vi "Process.vi"(8 "error in":errorcluster, 11 "Instrument.Framework-Template in":refnum<class "Instrument.Framework-Template.lvclass">) -> (0 "error out":errorcluster, 3 "Instrument.Framework-Template out":refnum<class "Instrument.Framework-Template.lvclass">)   [LabVIEW 2019, in "Instrument.Framework-Template.lvclass"]
doc: "---------------------------------------------------------------\nJKI State Machine Objects™\nhttp://jki.net/state-machine-objects/\nCopyright (C) 2005-2015, JKI <info@jki.net>\nALL RIGHTS RESERVED"
uses:
  Instrument.Framework-Template.lvclass
  <userlib>/LevyLab/Instrument Framework/Instrument/Instrument.lvclass
  <userlib>/LevyLab/RemoteControl/RemoteControl/Typedefs/Message--Cluster.ctl
  <userlib>/LevyLab/RemoteControl/RemoteControl/RemoteControl.lvclass
  Typedefs/PrivateEvents--Framework-Template.MessageToProcess.ctl
  C:/Program Files (x86)/National Instruments/LabVIEW 2019/user.lib/LevyLab/Instrument Framework/Instrument Types/SCPI/Instrument.SCPI.lvclass
  C:/Program Files (x86)/National Instruments/LabVIEW 2019/user.lib/LevyLab/Instrument Framework/Instrument/Instrument.lvclass
  C:/Program Files (x86)/National Instruments/LabVIEW 2019/vi.lib/JKI/JKI SMO/SMO/SMO.lvclass
  <userlib>/LevyLab/Debug/Debug.lvlib
  <userlib>/LevyLab/Instrument Framework/Instrument/API/Instrument.sendMessageToProcess (variant).vi
  <vilib>/JKI/JKI SMO/SMO/SMO.lvclass
  <userlib>/LevyLab/Instrument Framework/Instrument Types/SCPI/Instrument.SCPI.lvclass
panel:
  out "Status":string
  out "State History":string
  # "Instrument.Framework-Template"
  # "Framework-Template"
  # "For instructions on how to use the JKI State Machine Objects, examples and video tutorials, visit:\nhttp://jki.net/state-machine-objects/\n\nJKI State Machine Objects™\nhttp://jki.net/state-machine-objects/\nCopyright (C) 2005-2015, JKI <info@jki.net>\nALL RIGHTS RESERVED"
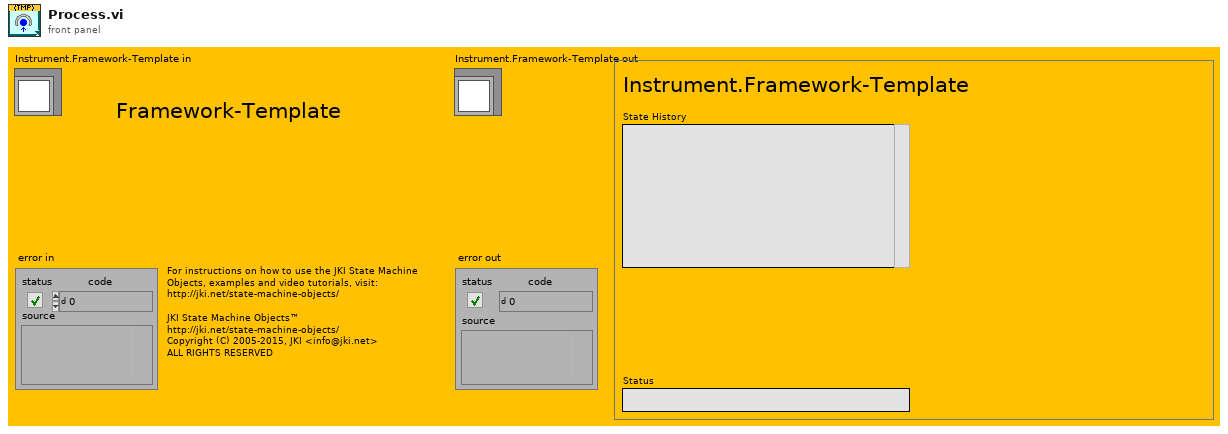
[diagram p1: front panel]
types:
  T1 = enum32{"invalid app kind", "Development System", "Run Time System", "Student Edition", "Embedded LabVIEW", "Evaluation", "Custom"}
  T2 = enum32{"Invalid", "Standard", "Closed", "Hidden", "Minimized", "Maximized"}
  T3 = typedef "RemoteControl.lvclass/Message--Cluster.ctl" = cluster{"Command":string, "Data":variant, "ID":string}
  T4 = typedef "Instrument.Framework-Template.lvclass/PrivateEvents--Framework-Template.MessageToProcess.ctl" = cluster{"Message":T5}
  T5 = typedef "RemoteControl.lvlib/RemoteControl.lvclass/Message--Cluster.ctl" = cluster{"Command":string, "Data":variant, "ID":string}
  T6 = cluster{"Core":cluster{"Current VI Reference":refnum<vi>, "Close Panel on Exit?":bool, "Last Error":cluster{"error":errorcluster, "previous state":string, "remaining states":string}, "Shutdown?":bool}, "SelfRef":refnum<class "Instrument.Framework-Template.lvclass">, "HAL":refnum<class "HAL.lvclass">, "Running Step":i32, "sequence":string[], "MessageToProcess":T4, "UI Behavior":string, "wait":u32}
  T7 = cluster{"Current VI Reference":refnum<vi>, "Close Panel on Exit?":bool, "Last Error":cluster{"error":errorcluster, "previous state":string, "remaining states":string}, "Shutdown?":bool}
  T8 = typedef "Debug.lvlib/Attribute.Debug.lvclass/DebugBehavior.ctl" = enum16{"Normal", "Debug"}
  T9 = typedef "SMO.lvclass/Protected Events.ctl" = cluster{"StopProcesses":refnum<user-event>, "AbortProcesses":refnum<user-event>, "Config Changed":refnum<user-event>, "Dependency":refnum<user-event>}
  T10 = typedef "Instrument.Framework-Template.lvclass/Instrument.Framework-Template.getAll--Cluster.ctl" = cluster{"Levy 1":dbl, "Logger SMO":dbl, "SMO Boolean":bool, "SMO String":string}
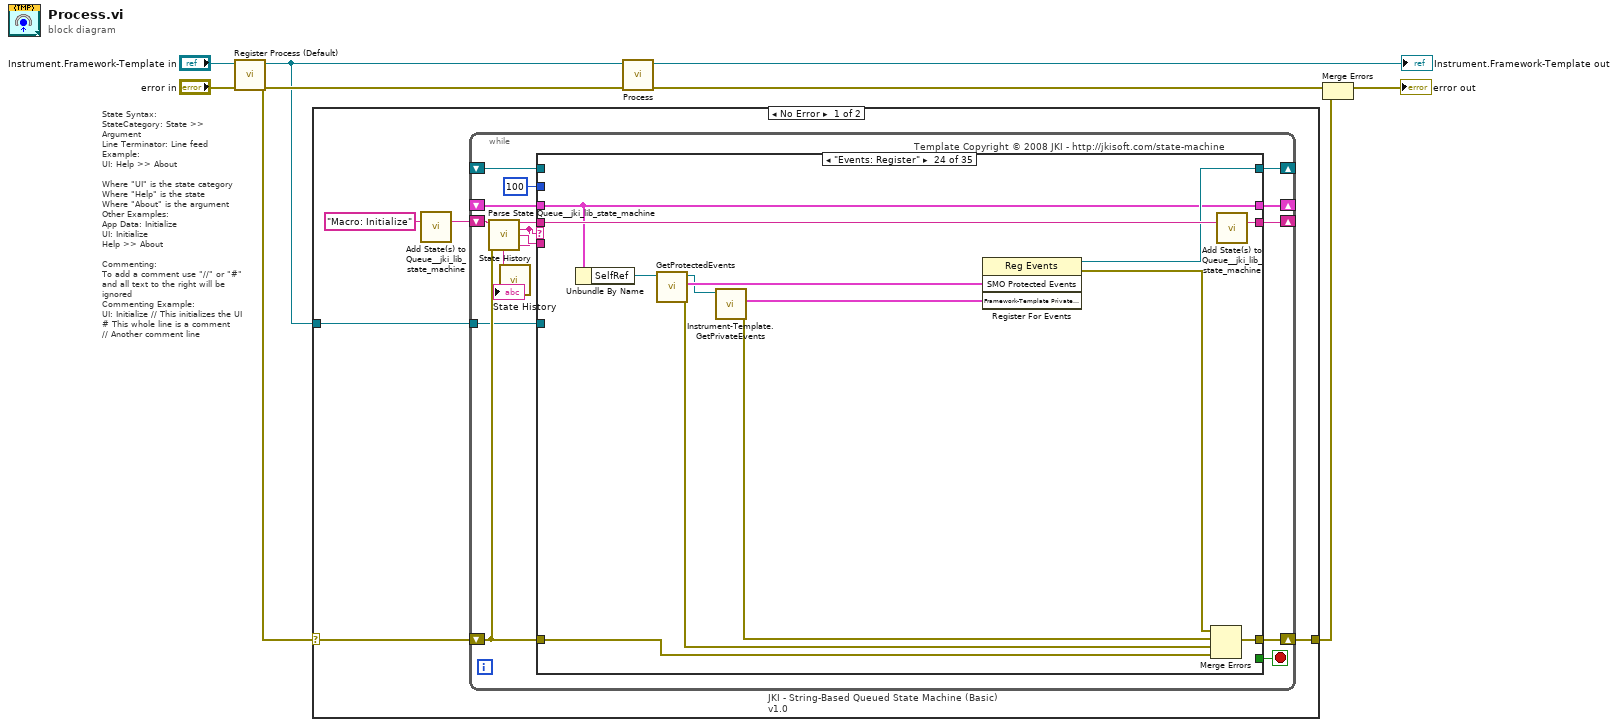
[diagram p0: block diagram]
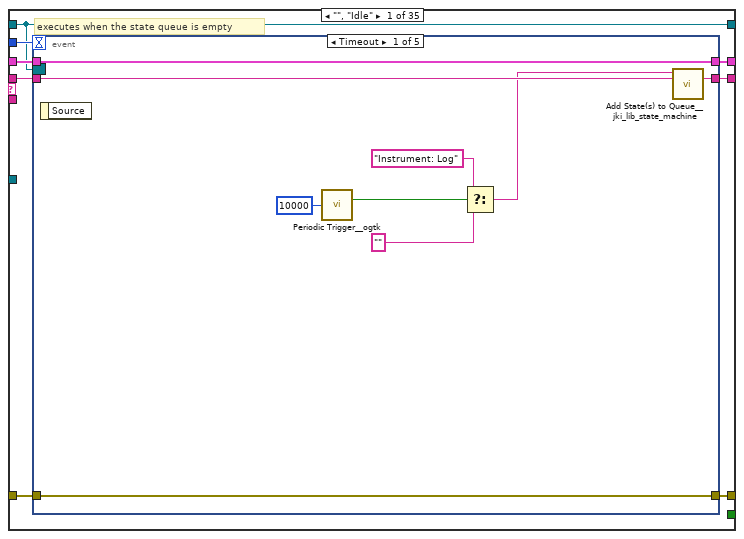
[diagram p2: hidden frame]
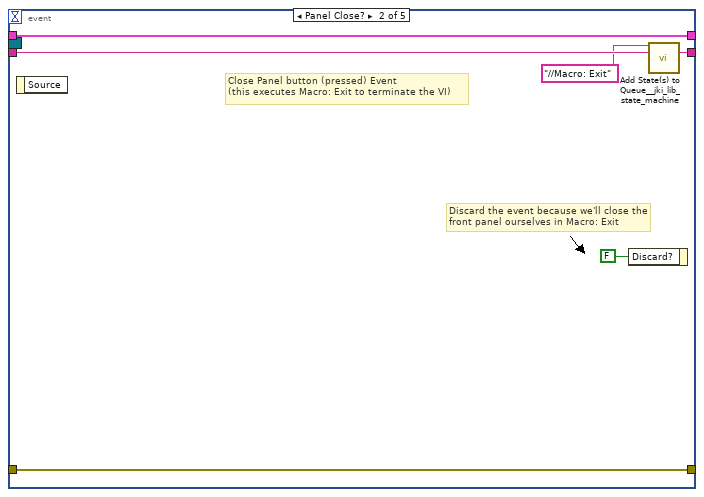
[diagram p3: hidden frame]
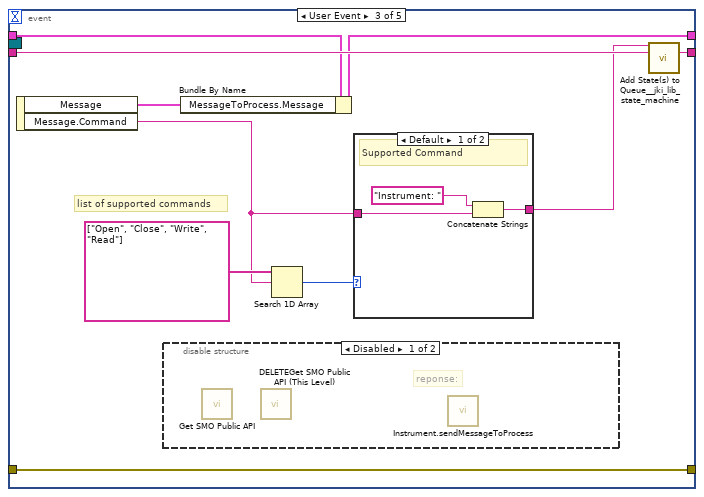
[diagram p4: hidden frame]
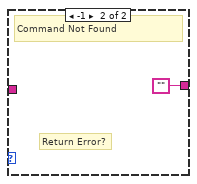
[diagram p6: hidden frame]
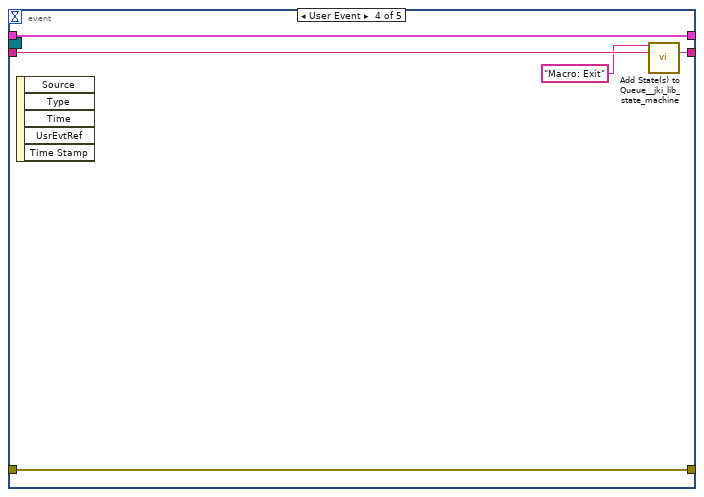
[diagram p7: hidden frame]
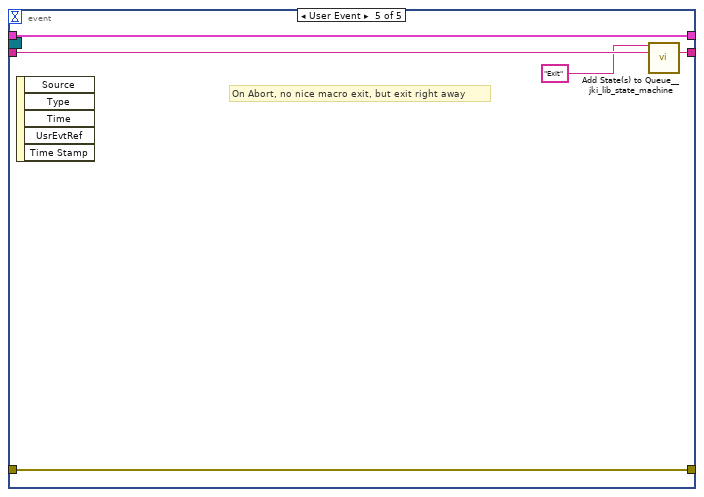
[diagram p8: hidden frame]
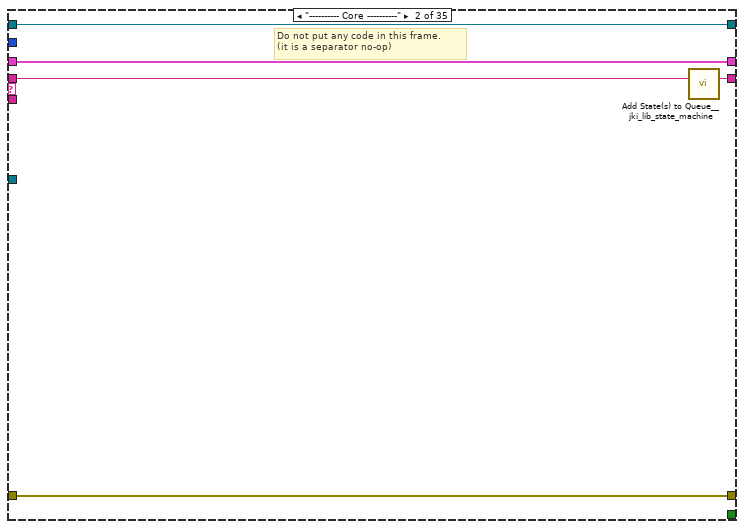
[diagram p9: hidden frame]
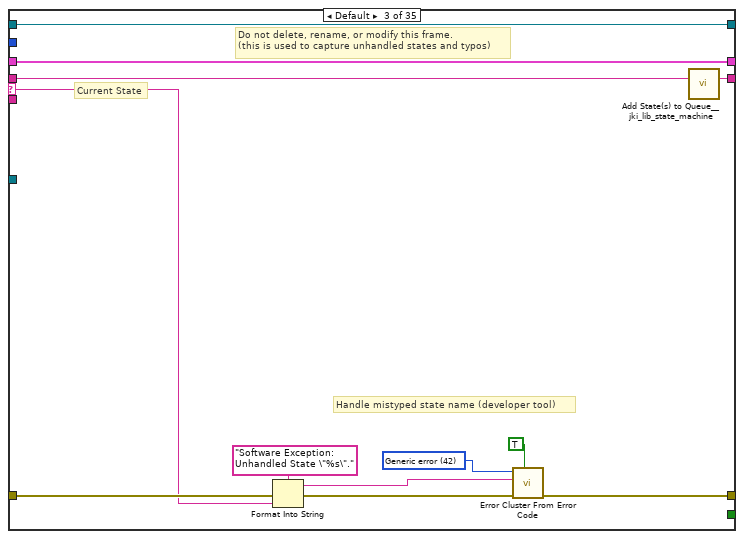
[diagram p10: hidden frame]
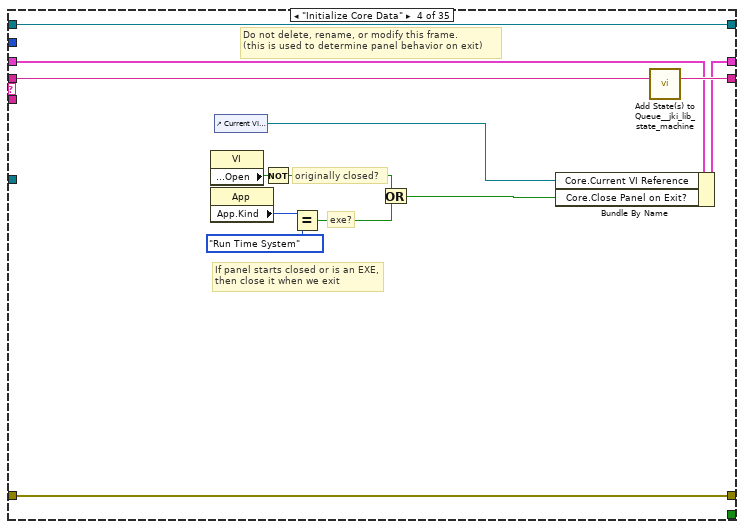
[diagram p11: hidden frame]
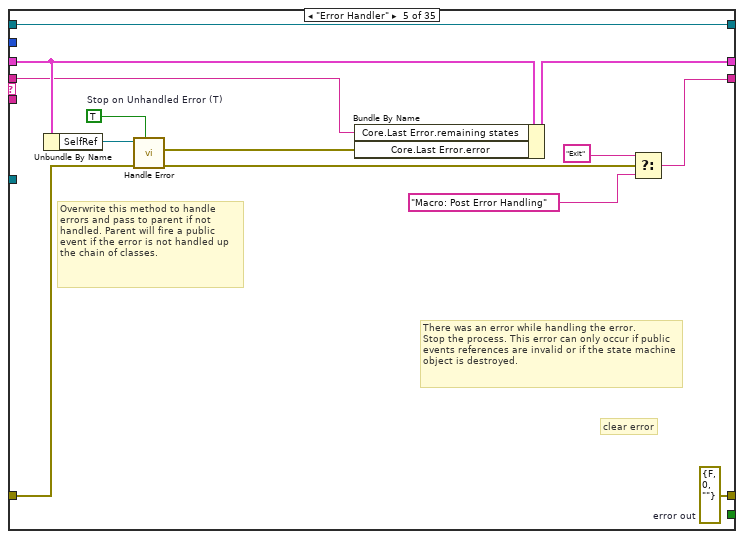
[diagram p12: hidden frame]
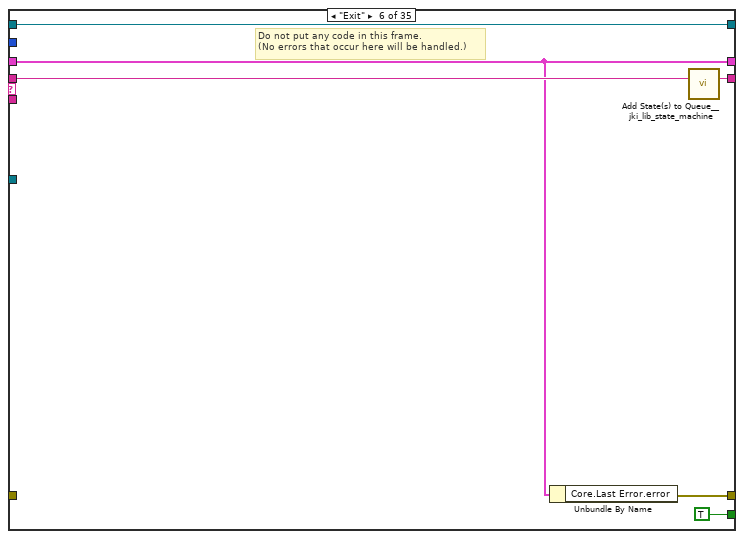
[diagram p13: hidden frame]
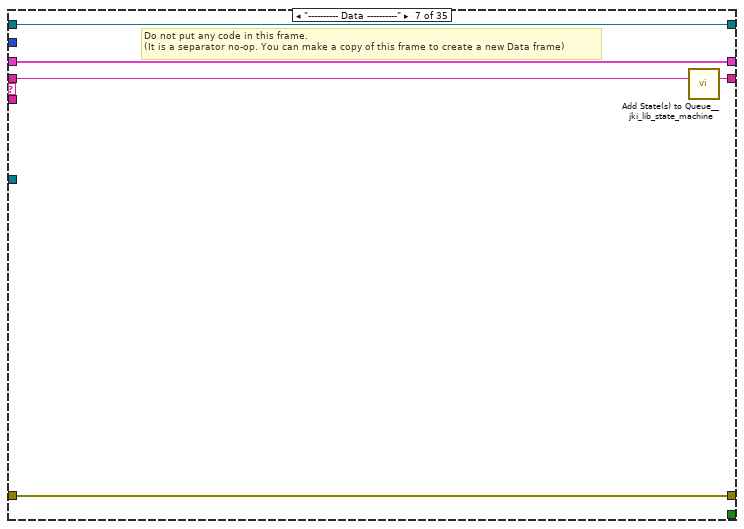
[diagram p14: hidden frame]
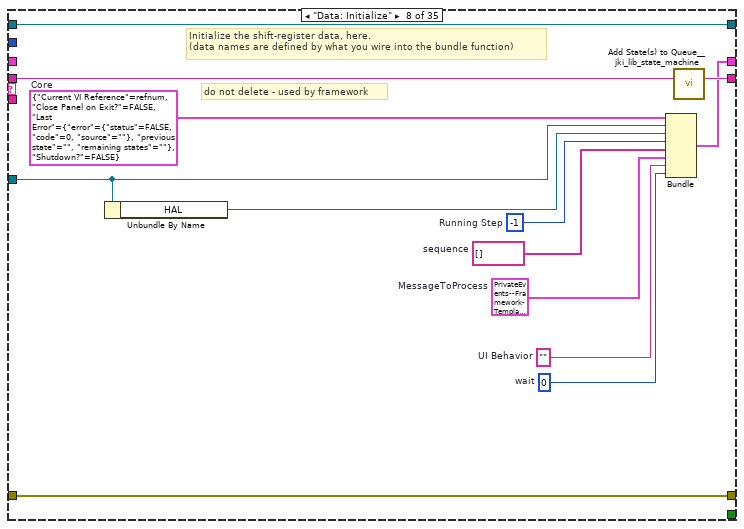
[diagram p15: hidden frame]
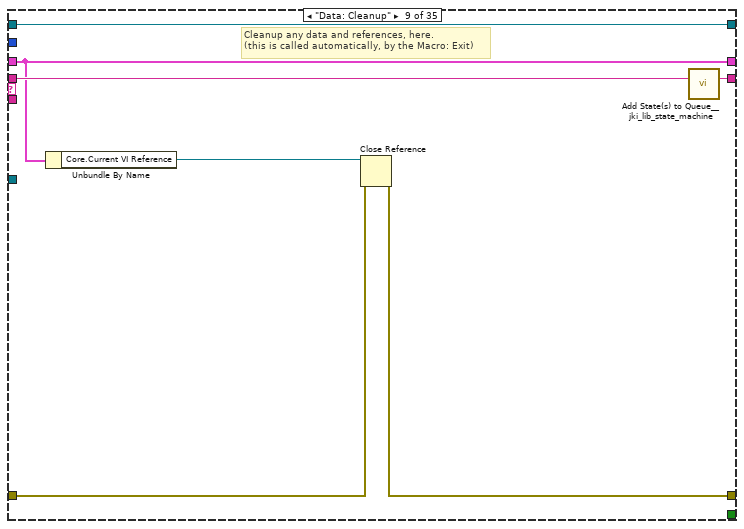
[diagram p16: hidden frame]
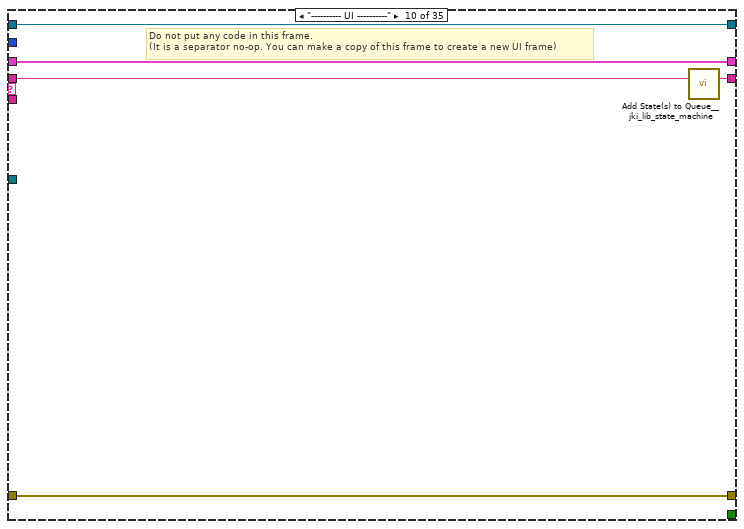
[diagram p17: hidden frame]
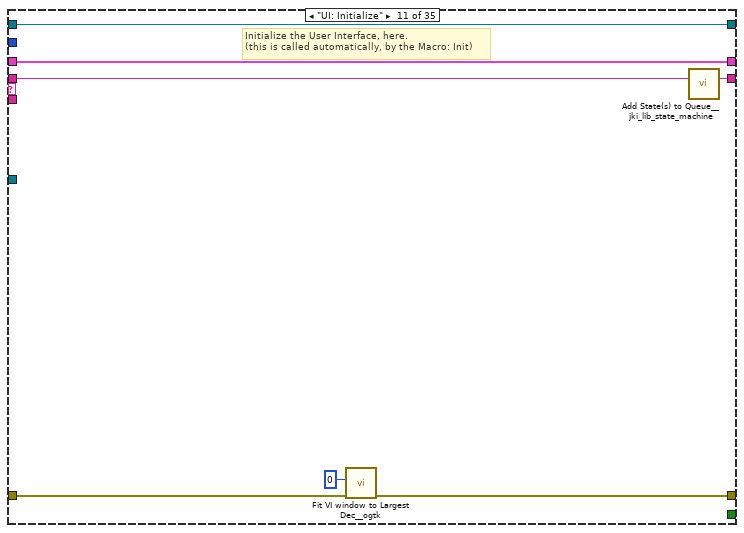
[diagram p18: hidden frame]
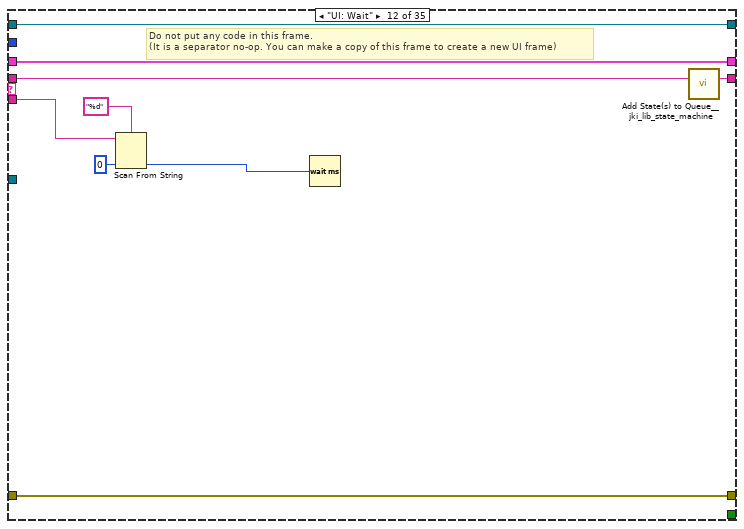
[diagram p19: hidden frame]
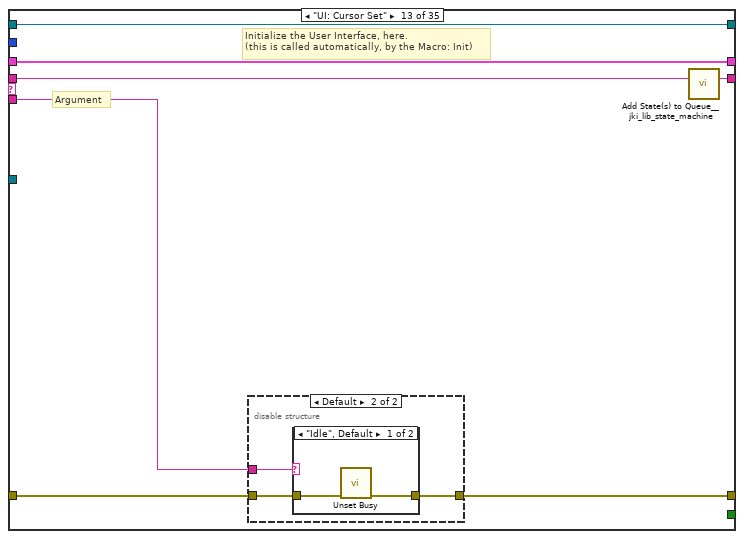
[diagram p20: hidden frame]
diagram:
  # "State Syntax:\nStateCategory: State >> Argument\nLine Terminator: Line feed\nExample:\nUI: Help >> About\n\nWhere \"UI\" is the state category\nWhere \"Help\" is the state\nWhere \"About\" is the argument\nOther Examples:\nApp Data: Initialize\nUI: Initialize\nHelp >> About\n\nCommenting:\nTo add a comment use \"//\" or \"#\" and all text to the right will be ignored\nCommenting Example:\nUI: Initialize // This initializes the UI\n# This whole line is a comment\n// Another comment line"
  n1 = call <vilib>:"Register Process (Default).vi"("error in (no error)"="error in", "SMO"="Instrument.Framework-Template in") -> ("error out"=w5:errorcluster, "SelfRef"=w4:refnum<class "Instrument.Framework-Template.lvclass">)  [unwired: 8 in]
  n2 = case shown="No Error" w5 {
    selector: w5 -> [w10 w455]
    tunnel: w4 -> [w11 _]
    tunnel: [w9 w455] -> w1
    frame No Error {
      n3 = call <vilib>:"Add State(s) to Queue__jki_lib_state_machine.vi"("State(s) in (\"\")"="Macro: Initialize") -> ("States Out"=w13:string)  [unwired: 14 in]
      n4 = while "JKI - String-Based Queued State Machine (Basic) v1.0" {
        shift-right: [w22] -> _
        shift-left: _ -> [w21]
        shift-right: [w25] -> w9
        shift-left: w10 -> [w19]
        shift-right: [w24] -> _
        shift-left: w13 -> [w26]
        tunnel: w11 -> [w18]
        shift-right: [w17] -> _
        shift-left: _ -> [w16]
        stop <- w23 stop-if-true
        # "Template Copyright © 2008 JKI - http://jkisoft.com/state-machine"
        n5 = call <vilib>:"Parse State Queue__jki_lib_state_machine.vi"("State Queue"=w26, "Error In (no error)"=w19) -> ("Remaining States"=w28:string, "Current State"=w15:string, "Arguments"=w27:string)  [unwired: 11 in]
        n6 = call <userlib>:"State History.vi"("Current State"=w15) -> ("History"=→"State History":string)  [unwired: 10 in]
        n7 = case shown="\"Events: Register\"" w15 {
          selector: w15 -> [_ _ w82 _ _ _ _ _ _ _ _ _ _ _ _ _ _ _ _ _ _ _ _ _ _ _ _ _ _ _ _ _ _ _ _]
          tunnel: w28 -> [w36 w80 w86 w105 w110 w124 w129 w142 w149 w154 w161 w170 w177 w193 w225 w234 w246 w267 w282 w304 w309 w320 w325 w338 w344 w352 w361 w370 w380 w389 w404 w424 w429 w435 w454]
          tunnel: w27 -> [_ _ _ _ _ _ _ _ _ _ _ w162 w171 w187 _ _ _ _ _ _ _ _ _ _ _ _ _ _ _ _ _ _ _ w430 w438]
          tunnel: w21 -> [w34 w77 w84 w96 w114 w120 w126 _ w144 w151 w159 w167 w175 w189 w222 w231 w236 w257 w271 w289 w306 w317 w322 w331 w342 w347 w357 w366 w376 w385 w400 w420 w425 w431 w444]
          tunnel: [w33 w78 w88 w102 w115 w119 w127 w132 w145 w152 w156 w168 w172 w190 w223 w226 w244 w265 w270 w292 w307 w311 w323 w334 w340 w349 w353 w365 w375 w384 w394 w418 w426 w432 w446] -> w25
          tunnel: w19 -> [w32 w78 w87 w102 w116 _ w127 w132 w146 w152 w155 w168 w173 w191 w223 w226 w244 w265 w269 w292 w307 w312 w323 w328 w340 w349 w356 w364 w374 w383 w398 w413 w426 w432 w440]
          tunnel: [w35 w79 w85 w104 w106 w123 w128 w141 w148 w153 w160 w169 w176 w192 w224 w233 w245 w266 w281 w303 w308 w319 w324 w337 w343 w351 w360 w369 w379 w388 w403 w423 w428 w434 w453] -> w24
          tunnel: [_ _ _ _ _ TRUE _ _ _ _ _ _ _ _ _ _ _ _ _ _ _ _ _ _ _ _ _ _ _ _ _ _ _ _ _] -> w23
          tunnel: [w31 w77 w84 w103 w113 w120 w126 w140 w144 w151 w159 w167 w175 w189 w222 w231 w237 w258 w272 w290 w306 w317 w322 w331 w342 w348 w358 w367 w377 w386 w401 w421 w425 w431 w443] -> w22
          tunnel: 100 ("Timeout") -> [w30 _ _ _ _ _ _ _ _ _ _ _ _ _ _ _ _ _ _ _ _ _ _ _ _ _ _ _ _ _ _ _ _ _ _]
          tunnel: w18 -> [_ _ _ _ _ _ _ w133 _ _ _ _ _ _ _ _ _ _ _ _ _ _ _ _ _ _ _ _ _ _ _ _ _ _ _]
          tunnel: [w29 w76 w81 w93 w118 w121 w125 w139 w143 w150 w158 w166 w174 w186 w221 w232 w243 w264 w280 w298 w305 w318 w321 w336 w341 w350 w359 w368 w378 w387 w402 w422 w427 w433 w452] -> w17
          tunnel: w16 -> [w29 w76 w81 w93 w118 w121 w125 w139 w143 w150 w158 w166 w174 w186 w221 w232 w243 w264 w280 w298 w305 w318 w321 _ w341 w350 w359 w368 w378 w387 w402 w422 w427 w433 w452]
          frame "", "Idle" {
            # "executes when the state queue is empty"
            n8 = event shown="[0] Timeout" {
              selector: w29 -> [_ _ _ _ _]
              dyn-events: _ -> [_ _ _ _ _]
              timeout: w30 -> [_ _ _ _ _]
              tunnel: w36 -> [w45 w51 w61 w70 w75]
              tunnel: [w44 w50 w60 w69 w74] -> w35
              tunnel: w34 -> [w42 w48 w53 w67 w72]
              tunnel: [w43 w49 w59 w68 w73] -> w33
              tunnel: w32 -> [w43 w49 w59 w68 w73]
              tunnel: [w42 w48 w54 w67 w72] -> w31
              event Timeout {
                n9 = event-data() -> ()  [unwired: 1 in, 1 out]
                n10 = call <userlib>:"Periodic Trigger__ogtk.vi"("time (ms)"=u32 10000) -> ("Triggered"=w39:bool)  [unwired: 12 in, 2 out]
                n11 = Select(t="Instrument: Log", s=w39, f="") -> (s? t:f=w40:string)
                n12 = call <vilib>:"Add State(s) to Queue__jki_lib_state_machine.vi"("State(s) in Front (\"\")"=w40, "State(s) in (\"\")"=w45) -> ("States Out"=w44:string)  [unwired: 13 in]
              }
              event Panel Close? {
                # "Discard the event because we'll close the front panel ourselves in Macro: Exit"
                # "Close Panel button (pressed) Event\n(this executes Macro: Exit to terminate the VI)"
                n13 = event-data() -> ()  [unwired: 1 in, 1 out]
                n14 = event-data("Discard?"=FALSE) -> ()  [unwired: 1 in, 1 out]
                n15 = call <vilib>:"Add State(s) to Queue__jki_lib_state_machine.vi"("State(s) in Front (\"\")"="//Macro: Exit", "State(s) in (\"\")"=w51) -> ("States Out"=w50:string)  [unwired: 13 in]
              }
              event User Event {
                # "list of supported commands"
                n16 = event-data() -> ("Message"=w52:T3, "Message.Command"=w55:string)  [unwired: 1 in]
                n17 = disable-structure shown="Disabled" {
                  frame Disabled {
                    # "reponse:"
                    n18 = call-dynamic "Get SMO Public API.vi"() -> ()  [unwired: 9 in, 3 out]
                    n19 = call-dynamic "DELETEGet SMO Public API (This Level).vi"() -> ()  [unwired: 9 in, 3 out]
                    n20 = call-poly <userlib>:"Instrument.sendMessageToProcess.vi"() -> ()  [unwired: 10 in, 2 out]
                  }
                  frame Enabled {
                  }
                }
                n21 = Bundle By Name(cluster=w53, "MessageToProcess.Message"=w52) -> (w54:T6)
                n22 = Search 1D Array(1D array=string[] ["Open", "Close", "Write", "Read"], element=w55) -> (index of element=w58:i32)  [unwired: 1 in]
                n23 = case shown="Default" w58 {
                  tunnel: [w64 ""] -> w56
                  tunnel: w55 -> [w63 _]
                  frame Default {
                    # "Supported Command"
                    n24 = Concatenate Strings("Instrument: ", w63) -> (w64:string)
                  }
                  frame -1 {
                    # "Return Error?"
                    # "Command Not Found"
                  }
                }
                n25 = call <vilib>:"Add State(s) to Queue__jki_lib_state_machine.vi"("State(s) in Front (\"\")"=w56, "State(s) in (\"\")"=w61) -> ("States Out"=w60:string)  [unwired: 13 in]
              }
              event User Event {
                n26 = event-data() -> ()  [unwired: 1 in, 5 out]
                n27 = call <vilib>:"Add State(s) to Queue__jki_lib_state_machine.vi"("State(s) in Front (\"\")"="Macro: Exit", "State(s) in (\"\")"=w70) -> ("States Out"=w69:string)  [unwired: 13 in]
              }
              event User Event {
                # "On Abort, no nice macro exit, but exit right away"
                n28 = event-data() -> ()  [unwired: 1 in, 5 out]
                n29 = call <vilib>:"Add State(s) to Queue__jki_lib_state_machine.vi"("State(s) in Front (\"\")"="Exit", "State(s) in (\"\")"=w75) -> ("States Out"=w74:string)  [unwired: 13 in]
              }
            }
          }
          frame "---------- Core ----------" {
            # "Do not put any code in this frame.\n(it is a separator no-op)"
            n30 = call <vilib>:"Add State(s) to Queue__jki_lib_state_machine.vi"("State(s) in (\"\")"=w80) -> ("States Out"=w79:string)  [unwired: 14 in]
          }
          frame Default {
            w91 = 42 items=["No error", "Argument error", "Memory is full", "Out of zone", "End of file", "File already open", "Generic file I/O error", "File not found", "File permission error", "Disk is full", "Duplicate path", "Too many files open", "System feature not enabled", "Resource file not found", "Cannot add resource", "Resource not found", "Image not found", "Image memory error", "Pen does not exist", "Config type invalid", "Config token not found", "Config parse error", "Config memory error", "Bad external code format", "Bad external code offset", "External code not present", "Null window", "Destroy window error", "Null menu", "Print aborted", "Bad print record", "Print driver error", "Windows error during printing", "Memory error during printing", "Print dialog error", "Generic print error", "Invalid device refnum", "Device not found", "Device parameter error", "Device unit error", "Cannot open device", "Device call aborted", "Generic error", "Cancelled by user", "Object ID too low", "Object ID too high", "Object not in heap", "Unknown heap", "Unknown object (invalid DefProc)", "Unknown object (DefProc not in table)", "Message out of range", "Invalid (null) method", "Unknown message", "Manager call not supported", "Bad address", "Network operation in progress", "Network operation timed out", "Connection is busy", "Network attribute not supported", "Network error", "Address in use", "System out of memory", "Connection aborted", "Connection refused", "Not connected", "Already connected", "Connection closed", "Initialization error (interapplication manager)", "Bad occurrence", "Wait on unbound occurrence handler", "Occurrence queue overflow", "Datalog type conflict", "Unused", "Unrecognized type (interapplication manager)", "Memory corrupt", "Failed to make temporary DLL", "Old CIN version", "Drag socket not found", "Failed to load drop-object", "Failed to register OLE object", "Failed to release OLE object", "Format specifier type mismatch", "Unknown format specifier", "Too few format specifiers", "Too many format specifiers", "Scan failed", "Newer CIN version", "Error converting to variant", "Runtime menu error", "Password tampered", "Variant attribute not found", "Incompatible variant data type", "Event data is not available", "Event Store is not present", "Occurrence is not found", "Event Queue is not created", "Event info is not available", "Refnum passed is NULL", "Error retrieving Class GUID", "Error retrieving CoClass GUID", "Error retrieving TypeLib GUID.", "Bad built application magic bytes.", "Specific driver is different from the specific driver associated with the Logical Name.", "There is no session opened to the class driver.", "Max Error", "MAX - Error with config objects", "MAX - Error loading configuration", "MAX - Group not supported"]
            # "Current State"
            # "Do not delete, rename, or modify this frame.\n(this is used to capture unhandled states and typos)"
            # "Handle mistyped state name (developer tool)"
            n31 = Format Into String(format string="Software Exception: Unhandled State \"%s\"." ("message"), error in=w87, w82) -> (resulting string=w90:string, error out=w89:errorcluster)  [unwired: 1 in]
            n32 = call <vilib>:"Error Cluster From Error Code.vi"("show call chain? (False)"=TRUE, "error in (no error)"=w89, "error message (\"\")"=w90, "error code (0)"=w91) -> ("error out"=w88:errorcluster)  [unwired: 5 in]
            n33 = call <vilib>:"Add State(s) to Queue__jki_lib_state_machine.vi"("State(s) in (\"\")"=w86) -> ("States Out"=w85:string)  [unwired: 14 in]
          }
          frame "Initialize Core Data" {
            # "Do not delete, rename, or modify this frame.\n(this is used to determine panel behavior on exit)"
            # "originally closed?"
            # "exe?"
            # "If panel starts closed or is an EXE, then close it when we exit"
            n34 = property class="VI"() -> ("Front Panel.Open"=w101:bool)  [unwired: 2 in, 2 out]
            n35 = property class="App"() -> ("App.Kind"=w100:T1)  [unwired: 2 in, 2 out]
            n36 = control-ref of="Current VI Reference"() -> (w94:refnum<vi>)
            n37 = Not(x=w101) -> (.not. x?=w98:bool)
            n38 = Equal?(x=w100, y=T1."Run Time System" ("Application:Kind")) -> (x = y?=w97:bool)
            n39 = Or(x=w98, y=w97) -> (x .or. y?=w95:bool)
            n40 = Bundle By Name(cluster=w96, "Core.Current VI Reference"=w94, "Core.Close Panel on Exit?"=w95) -> (w103:T6)
            n41 = call <vilib>:"Add State(s) to Queue__jki_lib_state_machine.vi"("State(s) in (\"\")"=w105) -> ("States Out"=w104:string)  [unwired: 14 in]
          }
          frame "Error Handler" {
            w111 = TRUE  # Stop on Unhandled Error (T)
            w115 = errorcluster {"status"=FALSE, "code"=0, "source"=""}  # error out
            # "clear error"
            # "There was an error while handling the error.\nStop the process. This error can only occur if public events references are invalid or if the state machine object is destroyed."
            # "Overwrite this method to handle errors and pass to parent if not handled. Parent will fire a public event if the error is not handled up the chain of classes."
            n42 = Unbundle By Name(w114) -> ("SelfRef"=w117:refnum<class "Instrument.Framework-Template.lvclass">)
            n43 = call-dynamic "Handle Error.vi"("Stop on Unhandled Error (T)"=w111, "error in"=w116, "SMO"=w117) -> ("handling error"=w107:errorcluster, "Unhandled error"=w112:errorcluster)  [unwired: 6 in, 1 out]
            n44 = Bundle By Name(cluster=w114, "Core.Last Error.remaining states"=w110, "Core.Last Error.error"=w112) -> (w113:T6)
            n45 = Select(t="Exit", s=w107, f="Macro: Post Error Handling") -> (s? t:f=w106:string)
          }
          frame "Exit" {
            # "Do not put any code in this frame.\n(No errors that occur here will be handled.)"
            n46 = Unbundle By Name(w120) -> ("Core.Last Error.error"=w119:errorcluster)
            n47 = call <vilib>:"Add State(s) to Queue__jki_lib_state_machine.vi"("State(s) in (\"\")"=w124) -> ("States Out"=w123:string)  [unwired: 14 in]
          }
          frame "---------- Data ----------" {
            # "Do not put any code in this frame.\n(It is a separator no-op. You can make a copy of this frame to create a new Data frame)"
            n48 = call <vilib>:"Add State(s) to Queue__jki_lib_state_machine.vi"("State(s) in (\"\")"=w129) -> ("States Out"=w128:string)  [unwired: 14 in]
          }
          frame "Data: Initialize" {
            w130 = u32 0  # wait
            w131 = ""  # UI Behavior
            w135 = T4 {"Message"={"Command"="", "Data"=variant(string ""), "ID"=""}}  # MessageToProcess
            w136 = string[] []  # sequence
            w137 = -1  # Running Step
            w138 = T7 {"Current VI Reference"=refnum, "Close Panel on Exit?"=FALSE, "Last Error"={"error"={"status"=FALSE, "code"=0, "source"=""}, "previous state"="", "remaining states"=""}, "Shutdown?"=FALSE}  # Core
            # "do not delete - used by framework"
            # "Initialize the shift-register data, here.\n(data names are defined by what you wire into the bundle function)"
            n49 = Unbundle By Name(w133) -> ("HAL"=w134:refnum<class "HAL.lvclass">)
            n50 = Bundle("Core"=w138, "SelfRef"=w133, "HAL"=w134, "Running Step"=w137, "sequence"=w136, "MessageToProcess"=w135, "UI Behavior"=w131, "wait"=w130) -> (w140:T6)  [unwired: 1 in]
            n51 = call <vilib>:"Add State(s) to Queue__jki_lib_state_machine.vi"("State(s) in (\"\")"=w142) -> ("States Out"=w141:string)  [unwired: 14 in]
          }
          frame "Data: Cleanup" {
            # "Cleanup any data and references, here.\n(this is called automatically, by the Macro: Exit)"
            n52 = Unbundle By Name(w144) -> ("Core.Current VI Reference"=w147:refnum<vi>)
            n53 = Close Reference(reference=w147, error in (no error)=w146) -> (error out=w145:errorcluster)
            n54 = call <vilib>:"Add State(s) to Queue__jki_lib_state_machine.vi"("State(s) in (\"\")"=w149) -> ("States Out"=w148:string)  [unwired: 14 in]
          }
          frame "---------- UI ----------" {
            # "Do not put any code in this frame.\n(It is a separator no-op. You can make a copy of this frame to create a new UI frame)"
            n55 = call <vilib>:"Add State(s) to Queue__jki_lib_state_machine.vi"("State(s) in (\"\")"=w154) -> ("States Out"=w153:string)  [unwired: 14 in]
          }
          frame "UI: Initialize" {
            # "Initialize the User Interface, here.\n(this is called automatically, by the Macro: Init)"
            n56 = call <userlib>:"Fit VI window to Largest Dec__ogtk.vi"("error in (no error)"=w155, "border spacing (2 px)"=0) -> ("error out"=w156:errorcluster)  [unwired: 4 in, 1 out]
            n57 = call <vilib>:"Add State(s) to Queue__jki_lib_state_machine.vi"("State(s) in (\"\")"=w161) -> ("States Out"=w160:string)  [unwired: 14 in]
          }
          frame "UI: Wait" {
            # "Do not put any code in this frame.\n(It is a separator no-op. You can make a copy of this frame to create a new UI frame)"
            n58 = Scan From String(format string="%d", input string=w162, default 1=u32 0 ("default value 1")) -> (output 1=w163:u32)  [unwired: 2 in, 3 out]
            n59 = Wait (ms)(milliseconds to wait=w163) -> ()  [unwired: 1 out]
            n60 = call <vilib>:"Add State(s) to Queue__jki_lib_state_machine.vi"("State(s) in (\"\")"=w170) -> ("States Out"=w169:string)  [unwired: 14 in]
          }
          frame "UI: Cursor Set" {
            # "Argument"
            # "Initialize the User Interface, here.\n(this is called automatically, by the Macro: Init)"
            n61 = disable-structure shown="Default" {
              disable-tunnel: w173 -> [w178 w181]
              disable-tunnel: [w178 w180] -> w172
              disable-tunnel: w171 -> [_ w179]
              frame condition #0 {
              }
              frame condition #1 (active) {
                n62 = case shown="\"Idle\", Default" w179 {
                  tunnel: w181 -> [w183 w185]
                  tunnel: [w182 w184] -> w180
                  frame "Idle", Default {
                    n63 = call <vilib>:"Unset Busy.vi"("error in (no error)"=w183) -> ("error out"=w182:errorcluster)  [unwired: 10 in]
                  }
                  frame "Busy" {
                    n64 = call <vilib>:"Set Busy.vi"("error in (no error)"=w185) -> ("error out"=w184:errorcluster)  [unwired: 9 in, 1 out]
                  }
                }
              }
            }
            n65 = call <vilib>:"Add State(s) to Queue__jki_lib_state_machine.vi"("State(s) in (\"\")"=w177) -> ("States Out"=w176:string)  [unwired: 14 in]
          }
          frame "UI: Front Panel State" {
            # "Argument"
            # "Set Front Panel Open or Closed\n(Usage: \"UI: Front Panel State >> Open|Close\")"
            n66 = Unbundle By Name(w189) -> ("Core.Current VI Reference"=w188:refnum<vi>)
            n67 = disable-structure shown="TARGET_TYPE==RT" {
              disable-tunnel: w191 -> [w197 w220]
              disable-tunnel: [w196 w220] -> w190
              disable-tunnel: w188 -> [w195 _]
              disable-tunnel: w187 -> [w194 _]
              frame condition #0 (active) {
                n68 = case shown="\"Close\"" w194 {
                  tunnel: w197 -> [w201 w214]
                  tunnel: [w203 w215] -> w196
                  tunnel: w195 -> [w202 w212]
                  frame "Open", Default {
                    n69 = property class="VI"(reference=w202, error in=w201) -> (reference out=w199:refnum<vi>, error out=w200:errorcluster, "FP.State"=w198:T2)
                    n70 = case shown="\"Closed\"" w198 {
                      tunnel: [w206 w209] -> w203
                      tunnel: w200 -> [w205 w209]
                      tunnel: w199 -> [w204 _]
                      frame "Closed" {
                        n71 = invoke class="VI" method="FP.Open"(reference=w204, error in=w205, "Activate"=TRUE, "State"=T2."Standard") -> (error out=w206:errorcluster)  [unwired: 1 in, 4 out]
                      }
                      frame Default {
                      }
                    }
                  }
                  frame "Close" {
                    n72 = property class="VI"(reference=w212, error in=w214) -> (reference out=w211:refnum<vi>, error out=w213:errorcluster, "FP.State"=w210:T2)
                    n73 = case shown="Default" w210 {
                      tunnel: [w216 w219] -> w215
                      tunnel: w213 -> [w216 w218]
                      tunnel: w211 -> [_ w217]
                      frame "Invalid", "Closed" {
                      }
                      frame Default {
                        n74 = invoke class="VI" method="FP.Close"(reference=w217, error in=w218) -> (error out=w219:errorcluster)  [unwired: 1 in, 2 out]
                      }
                    }
                  }
                }
              }
              frame condition #1 {
              }
            }
            n75 = call <vilib>:"Add State(s) to Queue__jki_lib_state_machine.vi"("State(s) in (\"\")"=w193) -> ("States Out"=w192:string)  [unwired: 14 in]
          }
          frame "---------- Macro ----------" {
            # "Do not put any code in this frame.\n(It is a separator no-op. You can make a copy of this frame to create a new Macro frame)"
            n76 = call <vilib>:"Add State(s) to Queue__jki_lib_state_machine.vi"("State(s) in (\"\")"=w225) -> ("States Out"=w224:string)  [unwired: 14 in]
          }
          frame "Macro: Initialize" {
            # "Initialization Macro\n(This is called once, when the VI starts)"
            n77 = call <vilib>:"Add State(s) to Queue__jki_lib_state_machine.vi"("State(s) in Front (\"\")"="Data: Initialize\nInitialize Core Data\nEvents: Register", "State(s) in (\"\")"="Process: Sync", "State(s) at Back (\"\")"="UI: Initialize\nUI: Front Panel State >> Close\nInstrument: Open\nMacro: Debug") -> ("States Out"=w229:string)  [unwired: 12 in]
            n78 = call <vilib>:"Add State(s) to Queue__jki_lib_state_machine.vi"("State(s) in Front (\"\")"=w229, "State(s) in (\"\")"=w234) -> ("States Out"=w233:string)  [unwired: 13 in]
          }
          frame "Macro: Post Error Handling" {
            # "Clear Last Error?"
            n79 = Unbundle By Name(w236) -> ("Core.Last Error.remaining states"=w238:string, "Core.Shutdown?"=w239:bool)
            n80 = Unbundle By Name(w236) -> ("Core.Last Error.error"=w242:errorcluster)
            n81 = case shown="False" FALSE {
              tunnel: w242 -> [w250 _]
              tunnel: [w250 _] -> w241
              frame False {
              }
              frame True {
              }
            }
            n82 = case shown="False" w239 {
              tunnel: w238 -> [w247 w249]
              tunnel: [w247 w248] -> w235
              frame False {
                # "These are the remaining states (at the moment the error occured). States can be altered according to business logic."
                # "NOT SHUTTING DOWN"
              }
              frame True {
                # "Developer can decide to alter the states but should be aware that during the shutdown process, there are certain states that must be run for the SMO to properly shut itself (and this process) down. As such, one can add states to perform additional clean-ups, but should append the remaining state to be executed."
                # "SHUTTING DOWN"
                n83 = call <vilib>:"Add State(s) to Queue__jki_lib_state_machine.vi"("State(s) in (\"\")"=w249) -> ("States Out"=w248:string)  [unwired: 14 in]
              }
            }
            n84 = Bundle By Name(cluster=w236, "Core.Last Error.error"=w241) -> (w237:T6)
            n85 = call <vilib>:"Add State(s) to Queue__jki_lib_state_machine.vi"("State(s) in Front (\"\")"=w235, "State(s) in (\"\")"=w246) -> ("States Out"=w245:string)  [unwired: 13 in]
          }
          frame "Macro: Run Sequence" {
            # "0,1,2,3,4,"
            # "5"
            # "Do not put any code in this frame.\n(It is a separator no-op. You can make a copy of this frame to create a new Macro frame)"
            n86 = Unbundle By Name(w257) -> ("sequence"=w253:string[], "Running Step"=w251:i32)
            n87 = Array Size(array=w253) -> (size(s)=w263:i32)
            n88 = Index Array(array=w253, index=w251) -> (element=w252:string)
            n89 = Greater Or Equal?(x=w263, y=w251) -> (x >= y?=w255:bool)
            n90 = Select(t=-1 ("Running Step"), s=w255, f=w251) -> (s? t:f=w262:i32)
            n91 = Bundle By Name(cluster=w257, "Running Step"=w262) -> (w258:T6)
            n92 = Select(t="Sequence: Status >> ...", s=w255, f="Idle //Check Event Structure\nMacro: Run Sequence" ("State(s) at Back (\"\")")) -> (s? t:f=w254:string)
            n93 = call <vilib>:"Add State(s) to Queue__jki_lib_state_machine.vi"("State(s) in Front (\"\")"=w252, "State(s) at Back (\"\")"=w254) -> ("States Out"=w256:string)  [unwired: 13 in]
            n94 = call <vilib>:"Add State(s) to Queue__jki_lib_state_machine.vi"("State(s) in Front (\"\")"=w256, "State(s) in (\"\")"=w267) -> ("States Out"=w266:string)  [unwired: 13 in]
          }
          frame "Macro: Debug" {
            # "exe?"
            # "If pane is an EXE, then close it when we exit"
            # "Macro: Debug\n(get debug behavior, determine UI and determine shutdown behavior)"
            n95 = Unbundle By Name(w271) -> ("Core.Close Panel on Exit?"=w274:bool, "SelfRef"=w279:refnum<class "Instrument.Framework-Template.lvclass">)
            n96 = property class="App"() -> ("App.Kind"=w277:T1)  [unwired: 2 in, 2 out]
            n97 = Equal?(x=w277, y=T1."Run Time System" ("Application:Kind")) -> (x = y?=w273:bool)
            n98 = call <userlib>:"Get Debug Mode.vi"("error in (no error)"=w269, "SMO"=w279) -> ("error out"=w270:errorcluster, "Behavior"=w278:T8)  [unwired: 7 in, 1 out]
            n99 = case shown="\"Normal\", Default" w278 {
              tunnel: [w283 w285] -> w275
              tunnel: w274 -> [w283 _]
              tunnel: w273 -> [_ w287]
              tunnel: [_ "UI: Front Panel State >> Open\nUI: Wait >> 1000"] -> w268
              frame "Normal", Default {
                # "respect core.close"
              }
              frame "Debug" {
                # "keep panel open\nunless exe"
                n100 = Or(x=w287, y=FALSE) -> (x .or. y?=w285:bool)
              }
            }
            n101 = Bundle By Name(cluster=w271, "Core.Close Panel on Exit?"=w275) -> (w272:T6)
            n102 = call <vilib>:"Add State(s) to Queue__jki_lib_state_machine.vi"("State(s) in Front (\"\")"=w268, "State(s) in (\"\")"=w282) -> ("States Out"=w281:string)  [unwired: 13 in]
          }
          frame "Macro: Exit" {
            # "Exit Macro\n(This is called once, when the VI exits)"
            n103 = Unbundle By Name(w289) -> ("Core.Close Panel on Exit?"=w302:bool)
            n104 = Select(t="UI: Front Panel State >> Close", s=w302, f="") -> (s? t:f=w300:string)
            n105 = Bundle By Name(cluster=w289, "Core.Shutdown?"=TRUE) -> (w290:T6)
            n106 = call <vilib>:"Add State(s) to Queue__jki_lib_state_machine.vi"("State(s) in Front (\"\")"="Data: Cleanup\nEvents: Unregister", "State(s) in (\"\")"="Process: Sync", "State(s) at Back (\"\")"="Exit") -> ("States Out"=w295:string)  [unwired: 12 in]
            n107 = call <vilib>:"Add State(s) to Queue__jki_lib_state_machine.vi"("State(s) in Front (\"\")"="Instrument: Close", "State(s) in (\"\")"=w300, "State(s) at Back (\"\")"=w295) -> ("States Out"=w299:string)  [unwired: 12 in]
            n108 = call <vilib>:"Add State(s) to Queue__jki_lib_state_machine.vi"("State(s) in Front (\"\")"=w299, "State(s) in (\"\")"=w304) -> ("States Out"=w303:string)  [unwired: 13 in]
          }
          frame "---------- Process ----------" {
            # "Template Separator\n(You can make a copy of, or modify, this frame)"
            n109 = call <vilib>:"Add State(s) to Queue__jki_lib_state_machine.vi"("State(s) in (\"\")"=w309) -> ("States Out"=w308:string)  [unwired: 14 in]
          }
          frame "Process: Sync" {
            n110 = Unbundle By Name(w317) -> ("SelfRef"=w313:refnum<class "Instrument.Framework-Template.lvclass">)
            n111 = call <vilib>:"WaitOnProcessSync.vi"("error in (no error)"=w312, "SMO"=w313) -> ("error out"=w311:errorcluster, "Don't run?"=w316:bool)  [unwired: 7 in, 1 out]
            n112 = Select(t="Data: Cleanup\nEvents: Unregister\nExit", s=w316, f="") -> (s? t:f=w310:string)
            n113 = call <vilib>:"Add State(s) to Queue__jki_lib_state_machine.vi"("State(s) in Front (\"\")"=w310, "State(s) in (\"\")"=w320) -> ("States Out"=w319:string)  [unwired: 13 in]
          }
          frame "---------- Events ----------" {
            # "Template Separator\n(You can make a copy of, or modify, this frame)"
            n114 = call <vilib>:"Add State(s) to Queue__jki_lib_state_machine.vi"("State(s) in (\"\")"=w325) -> ("States Out"=w324:string)  [unwired: 14 in]
          }
          frame "Events: Register" {
            n115 = Unbundle By Name(w331) -> ("SelfRef"=w332:refnum<class "Instrument.Framework-Template.lvclass">)
            n116 = call <vilib>:"GetProtectedEvents.vi"("SMO"=w332) -> ("error out"=w330:errorcluster, "SMO Protected Events"=w335:T9, "SMO out"=w329:refnum<class "Instrument.Framework-Template.lvclass">)  [unwired: 8 in]
            n117 = call "Instrument-Template.GetPrivateEvents.vi"("Instrument.Framework-Template in"=w329) -> ("error out"=w326:errorcluster, "Framework-Template Private Events"=w327:cluster{"MessageToProcess":refnum<user-event>})  [unwired: 8 in, 1 out]
            n118 = register-events(w335, w327) -> (reference out=w336:refnum<event-registration>, error out=w333:errorcluster)  [unwired: 2 in]
            n119 = Merge Errors(w333, w326, w330, w328) -> (w334:errorcluster)
            n120 = call <vilib>:"Add State(s) to Queue__jki_lib_state_machine.vi"("State(s) in (\"\")"=w338) -> ("States Out"=w337:string)  [unwired: 14 in]
          }
          frame "Events: Unregister" {
            n121 = Unregister For Events(event registration refnum=w341, error in=w340) -> (error out=w339:errorcluster)
            n122 = call <vilib>:"Clear Errors.vi"("error in (no error)"=w339) -> ()  [unwired: 5 in, 2 out]
            n123 = call <vilib>:"Add State(s) to Queue__jki_lib_state_machine.vi"("State(s) in (\"\")"=w344) -> ("States Out"=w343:string)  [unwired: 14 in]
          }
          frame "---------- Instrument ----------" {
            n124 = Unbundle By Name(w347) -> ("SelfRef"=w345:refnum<class "Instrument.Framework-Template.lvclass">, "HAL"=w346:refnum<class "HAL.lvclass">)
            n125 = Bundle By Name(cluster=w347, "SelfRef"=w345, "HAL"=w346) -> (w348:T6)
            n126 = call <vilib>:"Add State(s) to Queue__jki_lib_state_machine.vi"("State(s) in (\"\")"=w352) -> ("States Out"=w351:string)  [unwired: 14 in]
          }
          frame "Instrument: Open" {
            n127 = Unbundle By Name(w357) -> ("SelfRef"=w355:refnum<class "Instrument.Framework-Template.lvclass">)
            n128 = call-dynamic "Open Hardware.vi"("error in (no error)"=w356, "Instrument in"=w355) -> ("error out"=w353:errorcluster, "Instrument out"=w354:refnum<class "Instrument.Framework-Template.lvclass">)  [unwired: 8 in]
            n129 = Bundle By Name(cluster=w357, "SelfRef"=w354) -> (w358:T6)
            n130 = call <vilib>:"Add State(s) to Queue__jki_lib_state_machine.vi"("State(s) in (\"\")"=w361) -> ("States Out"=w360:string)  [unwired: 14 in]
          }
          frame "Instrument: Write" {
            n131 = Unbundle By Name(w366) -> ("SelfRef"=w363:refnum<class "Instrument.Framework-Template.lvclass">)
            n132 = call-dynamic "Write Hardware.vi"("error in (no error)"=w364, "Instrument in"=w363) -> ("error out"=w365:errorcluster, "Instrument out"=w362:refnum<class "Instrument.Framework-Template.lvclass">)  [unwired: 8 in]
            n133 = Bundle By Name(cluster=w366, "SelfRef"=w362) -> (w367:T6)
            n134 = call <vilib>:"Add State(s) to Queue__jki_lib_state_machine.vi"("State(s) in (\"\")"=w370) -> ("States Out"=w369:string)  [unwired: 14 in]
          }
          frame "Instrument: Read" {
            n135 = Unbundle By Name(w376) -> ("SelfRef"=w372:refnum<class "Instrument.Framework-Template.lvclass">)
            n136 = call-dynamic "Read Hardware.vi"("error in (no error)"=w374, "Instrument in"=w372) -> ("error out"=w375:errorcluster, "response"=w373:string, "Instrument out"=w371:refnum<class "Instrument.Framework-Template.lvclass">)  [unwired: 7 in]
            n137 = Bundle By Name(cluster=w376, "SelfRef"=w371, "MessageToProcess.Message.Data"=w373) -> (w377:T6)
            n138 = call <vilib>:"Add State(s) to Queue__jki_lib_state_machine.vi"("State(s) in (\"\")"=w380) -> ("States Out"=w379:string)  [unwired: 14 in]
          }
          frame "Instrument: Close" {
            n139 = Unbundle By Name(w385) -> ("SelfRef"=w382:refnum<class "Instrument.Framework-Template.lvclass">)
            n140 = call-dynamic "Close Hardware.vi"("error in (no error)"=w383, "Instrument in"=w382) -> ("error out"=w384:errorcluster, "Instrument out"=w381:refnum<class "Instrument.Framework-Template.lvclass">)  [unwired: 8 in]
            n141 = Bundle By Name(cluster=w385, "SelfRef"=w381) -> (w386:T6)
            n142 = call <vilib>:"Add State(s) to Queue__jki_lib_state_machine.vi"("State(s) in (\"\")"=w389) -> ("States Out"=w388:string)  [unwired: 14 in]
          }
          frame "Instrument: Do Something" {
            # "communicate with\nhardware"
            n143 = Unbundle By Name(w400) -> ("SelfRef"=w399:refnum<class "Instrument.Framework-Template.lvclass">, "MessageToProcess.Message.Data"=w397:variant, "MessageToProcess.Message.ID"=w392:string)
            n144 = call "Instrument-Template.doSomethingExample.vi"("error in (no error)"=w398, "Data"=w397, "Instrument.Framework-Template in"=w399) -> ("error out"=w393:errorcluster, "Data out"=w391:variant, "Instrument.Framework-Template out"=w396:refnum<class "Instrument.Framework-Template.lvclass">)  [unwired: 6 in]
            n145 = Empty String/Path?(string/path=w391) -> (empty?=w390:bool)
            n146 = case shown="False" w390 {
              tunnel: w396 -> [w409 w411]
              tunnel: [w406 w411] -> w395
              tunnel: [w405 w410] -> w394
              tunnel: w391 -> [w408 _]
              tunnel: w393 -> [w407 w410]
              tunnel: w392 -> [_ _]
              frame False {
                # "send data to\ninstrument:process.vi"
                n147 = call <userlib>:"setAllData.vi"("error in (no error)"=w407, "AllData"=w408, "Instrument in"=w409) -> ("error out"=w405:errorcluster, "Instrument out"=w406:refnum<class "Instrument.Framework-Template.lvclass">)  [unwired: 7 in]
              }
              frame True {
              }
            }
            n148 = Bundle By Name(cluster=w400, "SelfRef"=w395) -> (w401:T6)
            n149 = call <vilib>:"Add State(s) to Queue__jki_lib_state_machine.vi"("State(s) in (\"\")"=w404) -> ("States Out"=w403:string)  [unwired: 14 in]
          }
          frame "Instrument: Log" {
            # "THIS process.vi is responsible for logging data. Logging can be triggered in the timeout (as shown in this template proces.vi's tieout case) OR it could be triggered by data changes, or any other way you can device.\n\nThe code above will log ALL data. But you have the ability to log a subset, log some items on a different schedule, etc."
            n150 = Unbundle By Name(w420) -> ("SelfRef"=w416:refnum<class "Instrument.Framework-Template.lvclass">)
            n151 = call-dynamic "Get SMO Database Paths.vi"("error in (no error)"=w413, "Instrument.Framework-Template in"=w416) -> ("error out"=w414:errorcluster, "Paths"=w417:string, "Instrument.Framework-Template out"=w412:refnum<class "Instrument.Framework-Template.lvclass">)  [unwired: 7 in]
            n152 = Unbundle By Name(w412) -> ("Data"=w415:T10)
            n153 = call <userlib>:"Instrument.logToDatabase.vi"("error in (no error)"=w414, "Data"=w415, "Paths"=w417, "Instrument"=w412) -> ("error out"=w418:errorcluster, "Instrument out"=w419:refnum<class "Instrument.Framework-Template.lvclass">)  [unwired: 6 in]
            n154 = Bundle By Name(cluster=w420, "SelfRef"=w419) -> (w421:T6)
            n155 = call <vilib>:"Add State(s) to Queue__jki_lib_state_machine.vi"("State(s) in (\"\")"=w424) -> ("States Out"=w423:string)  [unwired: 14 in]
          }
          frame "---------- Sequence ----------" {
            n156 = call <vilib>:"Add State(s) to Queue__jki_lib_state_machine.vi"("State(s) in (\"\")"=w429) -> ("States Out"=w428:string)  [unwired: 14 in]
          }
          frame "Sequence: Status" {
            # "Sequence: Status\n(Use this frame to pass the status to the UI, this VI's UI, etc)"
            n157 = call <vilib>:"Add State(s) to Queue__jki_lib_state_machine.vi"("State(s) in (\"\")"=w435) -> ("States Out"=w434:string)  [unwired: 14 in]
            "Status" <- w430
          }
          frame "Sequence: Wait" {
            # "Sequence: Wait\n(Non-Blocking Wait)"
            # "F = repeat this state. wait\nT = go to next state. don't wait"
            n158 = Unbundle By Name(w444) -> ("Running Step"=w437:i32)
            n159 = call <userlib>:"Wait Logic.vi"("error in (no error)"=w440, "Time"=w438) -> ("error out"=w439:errorcluster, "Status String"=w436:string, "Trigger"=w441:bool)  [unwired: 6 in, 1 out]
            n160 = Increment(x=w437) -> (x+1=w451:i32)
            n161 = Select(t=w451, s=w441, f=w437) -> (s? t:f=w442:i32)
            n162 = Select(t=u32 0, s=w441, f=u32 100 ("milliseconds to wait")) -> (s? t:f=w448:u32)
            n163 = call <userlib>:"Wait (ms)__ogtk.vi"("error in (no error)"=w439, "milliseconds to wait"=w448) -> ("error out"=w446:errorcluster)  [unwired: 8 in, 1 out]
            n164 = Bundle By Name(cluster=w444, "Running Step"=w442) -> (w443:T6)
            n165 = call <vilib>:"Build State String with Arguments__JKI_lib_State_Machine.vi"("Arguments (\"\")"=w436, "State"="Sequence: Status") -> ("State with Arguments"=w445:string)  [unwired: 4 in]
            n166 = call <vilib>:"Add State(s) to Queue__jki_lib_state_machine.vi"("State(s) in Front (\"\")"=w445, "State(s) in (\"\")"=w454) -> ("States Out"=w453:string)  [unwired: 13 in]
          }
        }
      }
    }
    frame Error {
    }
  }
  n167 = call-parent "Process.vi"("error in"=w5, "Instrument"=w4) -> ("error out"=w2:errorcluster, "Instrument out"=→"Instrument.Framework-Template out":refnum<class "Instrument.Framework-Template.lvclass">)  [unwired: 8 in]
  n168 = Merge Errors(w2, w1) -> (→"error out":errorcluster)
